vi "create queue.vi"(8 "error in (no error)":errorcluster) -> (0 "error out":errorcluster, 3 "queue out":refnum<queue>)   [LabVIEW 2024]
doc: "The type of data that the queue will host is defined. The data type is a cluster containing a string for the status and a variant for the data."
uses:
  controls/State & Data Cluster.ctl
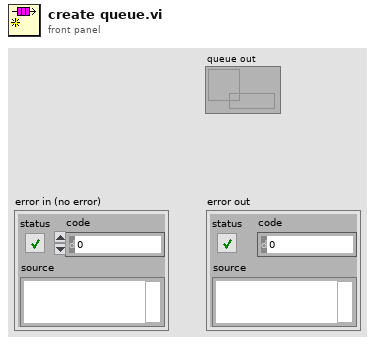
[diagram p1: front panel]
types:
  T1 = typedef "State & Data Cluster.ctl" = cluster{"State":string, "Data":variant}
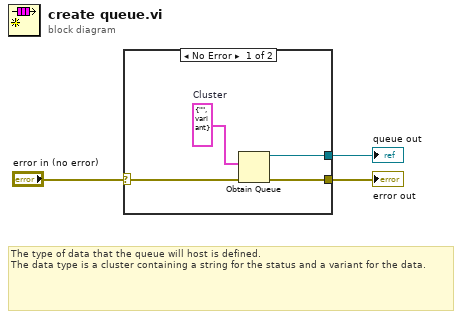
[diagram p0: block diagram]
diagram:
  # "The type of data that the queue will host is defined. \nThe data type is a cluster containing a string for the status and a variant for the data."
  n1 = case shown="No Error" "error in (no error)" {
    selector: "error in (no error)" -> [w4 w8]
    tunnel: [w7 w8] -> w3
    tunnel: [w6 _] -> w2
    frame No Error {
      w5 = T1 {"State"="", "Data"=variant}  # Cluster
      n2 = Obtain Queue(element data type=w5, error in (no error)=w4) -> (queue out=w6:refnum<queue>, error out=w7:errorcluster)  [unwired: 3 in, 1 out]
    }
    frame Error {
    }
  }
  "error out" <- w3
  "queue out" <- w2
